vi "Parse CSV From Disk.vi"(0 "File":path, 4 "Header Row?":bool=TRUE) -> (5 "Output Array":dbl[][](array[numeric]))   [LabVIEW 2012]
uses:
  <vilib>/Utility/file.llb/Read From Spreadsheet File (string).vi
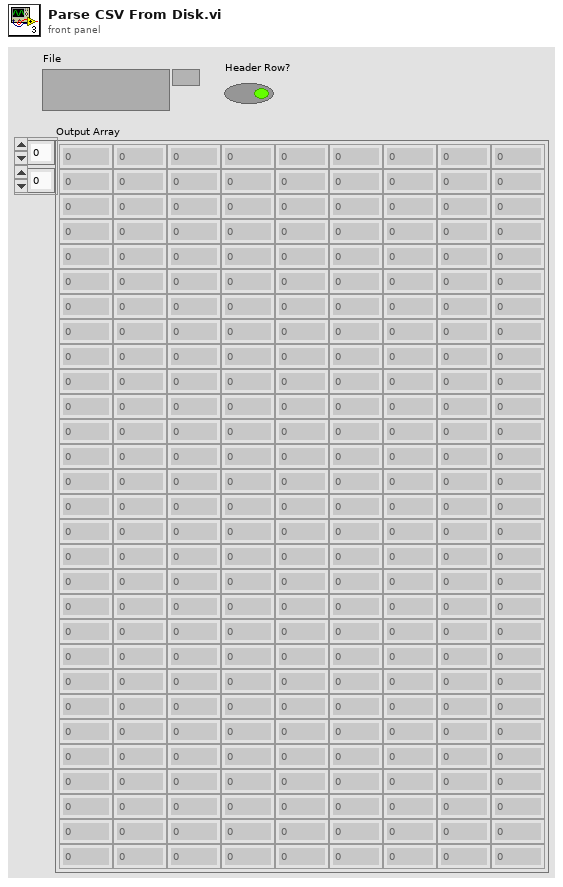
[diagram p1: front panel]
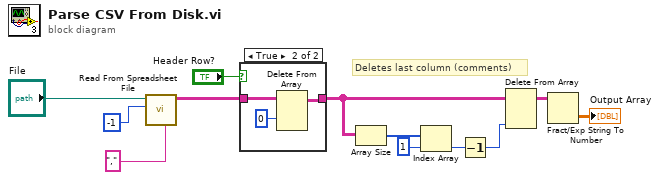
[diagram p0: block diagram]
diagram:
  # "Deletes last column (comments)"
  n1 = call-poly <vilib>:"Read From Spreadsheet File.vi"("delimiter (\\t)"="," ("delimiter (\\t)"), "number of rows (all:-1)"=-1, "file path (dialog if empty)"="File") -> ("all rows"=w10:string[][])  [unwired: 2 in, 6 out]
  n2 = case shown="True" "Header Row?" {
    tunnel: w10 -> [w13 w16]
    tunnel: [w13 w14] -> w2
    frame False {
    }
    frame True {
      n3 = Delete From Array(array=w16, index (row)=0) -> (array with subset deleted=w14:string[][])  [unwired: 2 in, 1 out]
    }
  }
  n4 = Array Size(array=w2) -> (size(s)=w7:i32[])
  n5 = Index Array "Index Array"(array=w7, index=1) -> (element=w5:i32)
  n6 = Decrement(x=w5) -> (x-1=w4:i32)
  n7 = Delete From Array(array=w2, index (col)=w4) -> (array with subset deleted=w3:string[][])  [unwired: 2 in, 1 out]
  n8 = Fract/Exp String To Number(string=w3) -> (number=→"Output Array":dbl[][])  [unwired: 3 in, 1 out]
